vi "Excel_Clear_Worksheet.vi"(0 "Excel._Worksheet":refnum<k7>, 5 "Excel.Shapes":refnum<k7>, 11 "error in (no error)":errorcluster) -> (15 "error out":errorcluster)   [LabVIEW 2020, in "NI_ReportGenerationToolkit.lvlib"]
uses:
  <vilib>/addons/_office/NI_ReportGenerationToolkit.lvlib
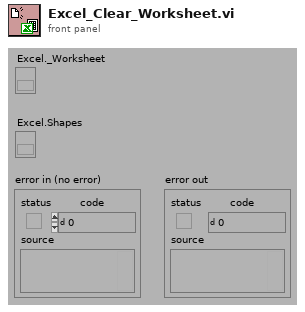
[diagram p1: front panel]
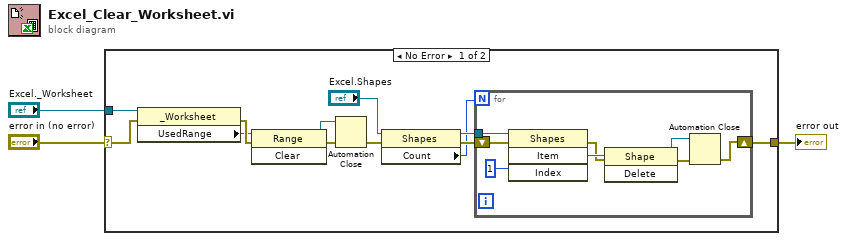
[diagram p0: block diagram]
diagram:
  n1 = case shown="No Error" "error in (no error)" {
    selector: "error in (no error)" -> [w4 w24]
    tunnel: [w15 w24] -> w3
    tunnel: "Excel._Worksheet" -> [w5 _]
    frame No Error {
      n2 = property class="_Worksheet"(reference=w5, error in=w4) -> (error out=w7:errorcluster, "UsedRange"=w6:refnum<k7>)  [unwired: 1 out]
      n3 = invoke class="Range" method="Clear"(reference=w6, error in=w7) -> (reference out=w9:refnum<k7>, error out=w8:errorcluster)  [unwired: 1 in, 1 out]
      n4 = Automation Close(3:w8, 5:w9) -> (0:w11:errorcluster)
      n5 = property class="Shapes"(reference="Excel.Shapes", error in=w11) -> (reference out=w13:refnum<k7>, error out=w14:errorcluster, "Count"=w12:i32)
      n6 = for {
        N: w12 -> [_]
        tunnel: w13 -> [w23]
        shift-right: [w17] -> w15
        shift-left: w14 -> [w18]
        n7 = invoke class="Shapes" method="Item"(reference=w23, error in=w18, "Index"=1) -> (error out=w21:errorcluster, "Item"=w22:refnum<k7>)  [unwired: 1 in, 2 out]
        n8 = invoke class="Shape" method="Delete"(reference=w22, error in=w21) -> (reference out=w19:refnum<k7>, error out=w20:errorcluster)  [unwired: 1 in, 1 out]
        n9 = Automation Close(3:w20, 5:w19) -> (0:w17:errorcluster)
      }
    }
    frame Error {
    }
  }
  "error out" <- w3
